vi "Constants.vi"() -> ()   [LabVIEW 2016]
panel:
  in  "Elevator":dbl=1.0
  in  "Agitator":dbl=-1.0
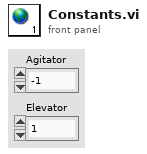
[diagram p1: front panel]
diagram:
